vi "Draw Markers.vi"(7 "Grid Size (10)":i32=10, 11 "Markers":bool[][](array[boolean])) -> (3 "Picture":picture)   [LabVIEW 2020, in "App.lvlib" / "MazeUI.lvclass"]
uses:
  MazeUI.lvclass
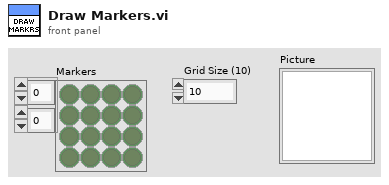
[diagram p1: front panel]
types:
  T1 = cluster{"Width":u16, "Style":enum32{"Solid", "Dash", "Dot", "DashDot", "DashDotDot"}}
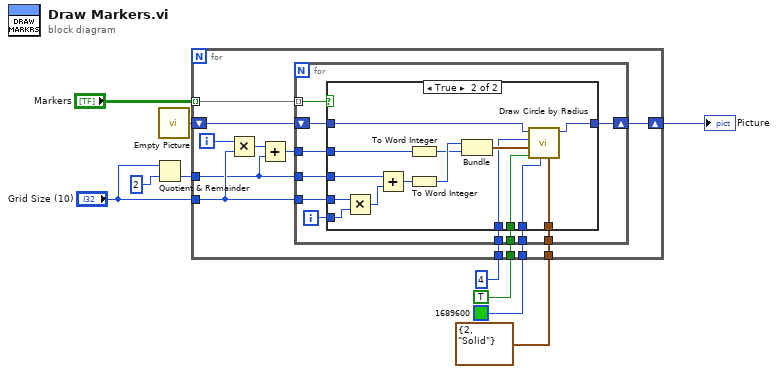
[diagram p0: block diagram]
diagram:
  n1 = Quotient & Remainder(x="Grid Size (10)", y=2) -> (floor(x/y)=w1:i32)  [unwired: 1 out]
  n2 = call "Empty Picture"() -> ("empty picture"=w10:picture)
  n3 = for {
    tunnel: T1 {"Width"=2, "Style"=enum."Solid"} ("pen") -> [w20]
    tunnel: u32 1689600 ("color(black)") -> [w19]
    tunnel: TRUE ("fill?(F)") -> [w18]
    tunnel: i16 4 ("radius") -> [w17]
    shift-right: [w21] -> w9
    shift-left: w10 -> [w22]
    tunnel: "Markers" -> [w16] mode=indexing
    tunnel: "Grid Size (10)" -> [w14]
    tunnel: w1 -> [w12]
    i -> [w15]
    n4 = Multiply(x=w15, y=w14) -> (x*y=w13:i32)
    n5 = Add(x=w13, y=w12) -> (x+y=w11:i32)
    n6 = for {
      shift-right: [w32] -> w21
      shift-left: w22 -> [w33]
      tunnel: w20 -> [w31]
      tunnel: w19 -> [w30]
      tunnel: w18 -> [w29]
      tunnel: w17 -> [w28]
      tunnel: w16 -> [w27] mode=indexing
      tunnel: w14 -> [w24]
      tunnel: w12 -> [w23]
      tunnel: w11 -> [w26]
      i -> [w25]
      n7 = case shown="True" w27 {
        tunnel: w33 -> [w34 w49]
        tunnel: [w34 w47] -> w32
        tunnel: w31 -> [_ w46]
        tunnel: w30 -> [_ w45]
        tunnel: w29 -> [_ w44]
        tunnel: w28 -> [_ w43]
        tunnel: w26 -> [_ w42]
        tunnel: w25 -> [_ w40]
        tunnel: w24 -> [_ w41]
        tunnel: w23 -> [_ w39]
        frame False {
        }
        frame True {
          n8 = Multiply(x=w41, y=w40) -> (x*y=w38:i32)
          n9 = Add(x=w39, y=w38) -> (x+y=w37:i32)
          n10 = To Word Integer(number=w42) -> (16bit integer=w35:i16)
          n11 = To Word Integer(number=w37) -> (16bit integer=w36:i16)
          n12 = Bundle(w36, w35) -> (w48:cluster{i16, i16})  [unwired: 1 in]
          n13 = call <vilib>:"Draw Circle by Radius.vi"("pen"=w46, "color(black)"=w45, "fill?(F)"=w44, "pixel center"=w48, "radius"=w43, "picture"=w49) -> ("new picture"=w47:picture)  [unwired: 5 in]
        }
      }
    }
  }
  "Picture" <- w9
